vi "Within Threshold.vi"(9 "Threshold":dbl, 10 "Center":dbl, 11 "Value":dbl) -> (3 "Within Threshold?":bool)   [LabVIEW 2018]
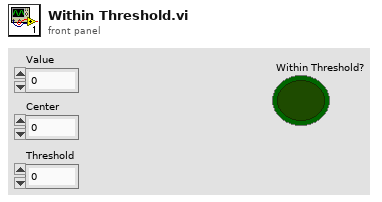
[diagram p1: front panel]
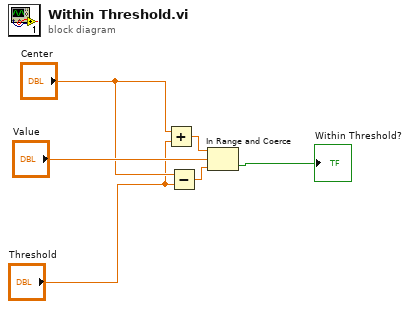
[diagram p0: block diagram]
diagram:
  n1 = Add(x="Center", y="Threshold") -> (x+y=w5:dbl)
  n2 = Subtract(x="Center", y="Threshold") -> (x-y=w4:dbl)
  n3 = In Range and Coerce(upper limit=w5, x="Value", lower limit=w4) -> (In Range?=→"Within Threshold?":bool)  [unwired: 1 out]
